vi "Timeout.vi"(1 "Done with Task?":bool, 2 "Timeout (ms)":u32) -> (0 "Timed Out?":bool)   [LabVIEW 2013]
panel:
  # "A vi for Dectecting if a Wait in a State Machine has Been Waiting \ntoo Long and Needs to Resend its Command"
  # "due to the issue with deciding when to initialize this, it looks like a FG inside..."
  # "...but it isn't so don't be decieved..."
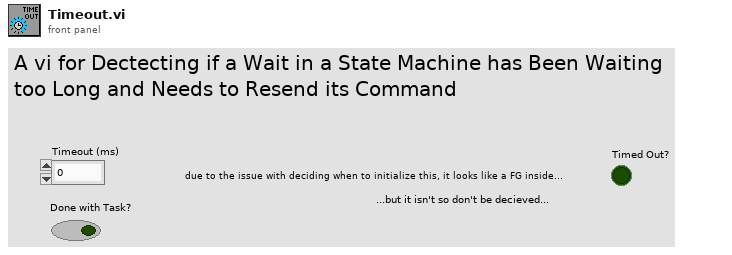
[diagram p1: front panel]
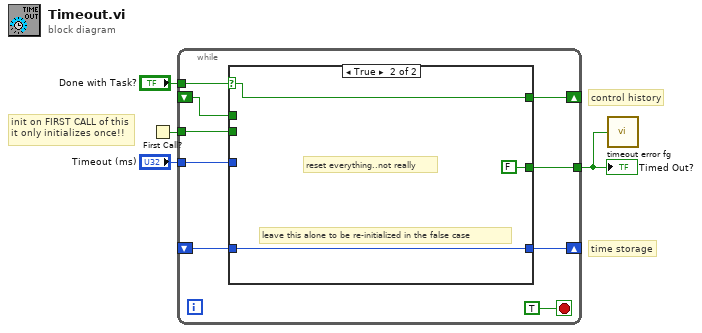
[diagram p0: block diagram]
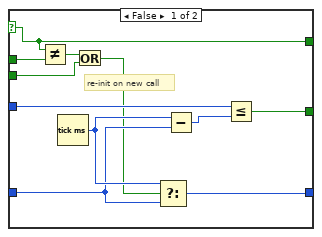
[diagram p2: hidden frame]
diagram:
  # "init on FIRST CALL of this\nit only initializes once!!"
  # "control history"
  # "time storage"
  n1 = First Call?() -> (First Call?: T/F=w1:bool)
  n2 = while {
    tunnel: "Timeout (ms)" -> [w10]
    shift-right: [w12] -> _
    shift-left: _ -> [w11]
    tunnel: [w9] -> w2
    shift-right: [w8] -> _
    shift-left: _ -> [w7]
    tunnel: "Done with Task?" -> [w6]
    tunnel: w1 -> [w5]
    stop <- TRUE stop-if-true
    n3 = case shown="True" w6 {
      selector: w6 -> [w18 w26]
      tunnel: [w22 w25] -> w12
      tunnel: w11 -> [w21 w25]
      tunnel: w10 -> [w20 _]
      tunnel: [w19 FALSE] -> w9
      tunnel: [w18 w26] -> w8
      tunnel: w7 -> [w17 _]
      tunnel: w5 -> [w14 _]
      frame False {
        # "re-init on new call"
        n4 = Not Equal?(x=w18, y=w17) -> (x != y?=w16:bool)
        n5 = Tick Count (ms)() -> (millisecond timer value=w24:u32)
        n6 = Or(x=w16, y=w14) -> (x .or. y?=w15:bool)
        n7 = Select(t=w24, s=w15, f=w21) -> (s? t:f=w22:u32)
        n8 = Subtract(x=w24, y=w21) -> (x-y=w23:u32)
        n9 = Less Or Equal?(x=w20, y=w23) -> (x <= y?=w19:bool)
      }
      frame True {
        # "leave this alone to be re-initialized in the false case"
        # "reset everything..not really"
      }
    }
  }
  "Timed Out?" <- w2
  n10 = call "timeout error fg.vi"("Timeout Error?"=w2) -> ()  [unwired: 2 out]
